vi "Average over data input 2.vi"() -> ()   [LabVIEW 2020]
uses:
  <vilib>/ptbypt/NI_PtbyPt.lvlib
panel:
  out "mean":dbl=-0.05816725885383049 format="%0.2f"
  out "Original function (blue), average value of function (red)":waveform(dbl)[](graph)=[{"t0"=timestamp(3778610283.2304187 s since 1904-01-01), "dt"=0.001, "Y"=array[1000 elements], "attributes"=variant("NI_ChannelName"=variant(string "Voltage"), "NI_UnitDescription"=variant(string "Volts"))}, {"t0"=timestamp(0 s since 1904-01-01), "dt"=0.001, "Y"=array[1000 elements]}]
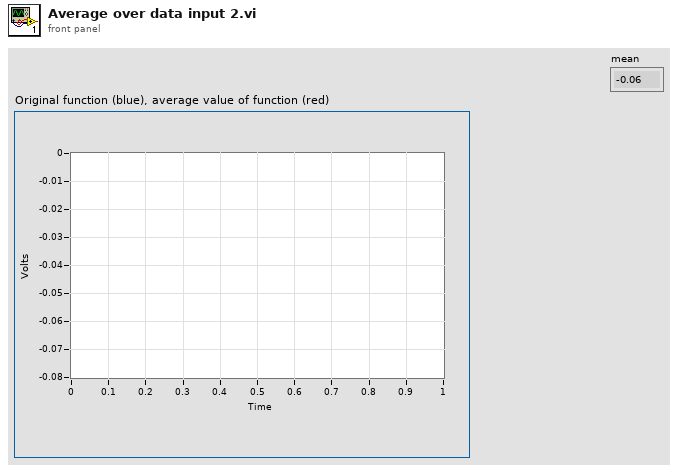
[diagram p1: front panel]
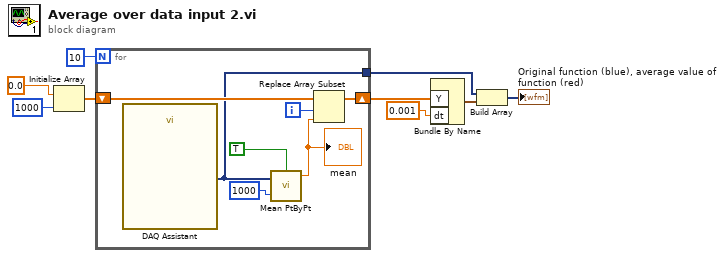
[diagram p0: block diagram]
diagram:
  n1 = Initialize Array(0.0 ("element"), 1000 ("dimension size")) -> (w7:dbl[])
  n2 = for {
    N: 10 -> [_]
    shift-right: [w13] -> w5
    shift-left: w7 -> [w14]
    tunnel: [w10] -> w2
    i -> [w12]
    n3 = call "DAQ Assistant"() -> ("data"=w10:dynamicdata)  [unwired: 16 in, 3 out]
    n4 = call <vilib>:"Mean PtByPt.vi"("x"=w10, "sample length"=1000, "initialize"=TRUE) -> ("mean"=w11:dbl)  [unwired: 1 in, 1 out]
    "mean" <- w11
    n5 = Replace Array Subset(array=w14, new element=w11, index=w12) -> (w13:dbl[])
  }
  n6 = Bundle By Name("Y"=w5, "dt"=0.001) -> (w4:waveform(dbl))  [unwired: 1 in]
  n7 = Build Array(w2, w4) -> (→"Original function (blue), average value of function (red)":dynamicdata[])
